vi "BonOMM-SAOMM.vi"() -> ()   [LabVIEW 2019] (continued)
            n4636 = call "PRAMMS-LISTENER.vi"("PRAMMS-COMM IN"=w2155, "Bool Refnum"=w2145, "MessageTypeArray"=w2152, "Signature"=w2144, "Error IN"=w2154, "ReadTimeOut"=4) -> ("Type"=w2147:string, "ByteArray"=w2151:u8[], "Received?"=w2153:bool)  [unwired: 4 in, 3 out]
            n4637 = flat-sequence {
              tunnel: w2153 -> [w2159]
              tunnel: w2151 -> [w2158]
              tunnel: w2147 -> [w2157]
              tunnel: w2139 -> [w2156]
              frame #0 {
                # "Lit toujours le socket prams et rafraichi l'image s'il s'agît d'une image ..."
                n4638 = case shown="Vrai" w2159 {
                  tunnel: w2157 -> [_ w2162]
                  tunnel: w2158 -> [_ w2161]
                  tunnel: w2156 -> [_ w2160]
                  frame False {
                  }
                  frame True {
                    n4639 = case shown="\"emtTelescopeServoLevel\"" w2162 {
                      selector: w2162 -> [w2164 _ _ _ _ _ _ _ _ _ _ _ _ _ _ _ _ _ _ _ _ _ _ w2454 _]
                      tunnel: w2161 -> [w2163 w2176 _ _ _ w2201 w2209 w2236 w2255 w2259 w2263 w2284 w2304 w2309 w2316 w2321 w2328 w2335 _ _ w2350 w2356 w2415 w2451 w2475]
                      tunnel: w2160 -> [_ _ _ _ _ _ _ _ _ _ _ _ _ _ _ _ _ _ _ _ _ _ _ _ w2463]
                      frame "Unknown", Default {
                        w2167 = "\r"
                        n4640 = Type Cast(type=w2167, x=w2163) -> (*(type *) &x=w2166:string)
                        n4641 = local read "Dump"() -> (w2169:string)
                        n4642 = Concatenate Strings(w2169, w2164, " : " ("string"), w2166, w2167) -> (→"Dump":string)
                      }
                      frame "emtError" {
                        # "Tableau d'exception qui ne causeront\npas l'affichage d'un message d'erreur."
                        n4643 = To Unsigned Long Integer(number=u32 0) -> (unsigned 32bit integer=w2178:u32)
                        n4644 = call-poly "SAOMM-EXTRACT-DATA.vi"("UINT32"=w2178, "Data"=w2176) -> ("Value"=w2173:u32)  [unwired: 10 in, 3 out]
                        n4645 = Search 1D Array(1D array=u32[] [64], element=w2173) -> (index of element=w2170:i32)  [unwired: 1 in]
                        n4646 = Less Than 0?(x=w2170) -> (x < 0?=w2171:bool)
                        n4647 = case shown="Vrai" w2171 {
                          tunnel: w2173 -> [_ w2182]
                          frame False {
                          }
                          frame True {
                            n4648 = Not Equal To 0?(x=w2182) -> (x != 0?=w2186:bool)
                            n4649 = case shown="Faux" w2186 {
                              tunnel: w2182 -> [_ w2193]
                              tunnel: ["Erreur reçu de PrAMS (code : indéfini)" w2189] -> w2187
                              frame False {
                              }
                              frame True {
                                n4650 = Number To Decimal String(number=w2193) -> (decimal integer string=w2192:string)  [unwired: 1 in]
                                n4651 = Concatenate Strings("Erreur reçu de PrAMS (code : ", w2192, ")") -> (w2189:string)
                              }
                            }
                            n4652 = local read "FIFO d'erreur"() -> (w2183:T7)
                            n4653 = call "Error_Format.vi"("FIFO IN"=w2183, "Error Code IN"=w2182, "Source"="PrAMS", "Comment"=w2187) -> ("FIFO OUT"=w2184:T7)  [unwired: 13 in, 2 out]
                            n4654 = local write "FIFO d'erreur"(w2184) -> ()
                          }
                        }
                        n4655 = To Long Integer(number=w2173) -> (32bit integer=w2174:i32)
                        n4656 = Negate(x=w2174) -> (-x=w2175:i32)
                        n4657 = local write "PrAMS-ACK"(w2175) -> ()
                        n4658 = local read "Nb_Error (PrAMS)"() -> (w2180:i32)
                        n4659 = Increment(x=w2180) -> (x+1=w2179:i32)
                        n4660 = local write "Nb_Error (PrAMS)"(w2179) -> ()
                        "PrAMS-Error" <- TRUE ("PrAMS-Error")
                      }
                      frame "emtAreYouThere" {
                      }
                      frame "emtAcknowledgment" {
                        n4661 = local read "Nb_ACK (PrAMS)"() -> (w2195:i32)
                        n4662 = Increment(x=w2195) -> (x+1=→"Nb_ACK (PrAMS)":i32)
                        "PrAMS-ACK" <- 1 ("PrAMS-ACK")
                      }
                      frame "emtClientType" {
                        # "Jamais reçu par BonOMM actuellement puisque BonOMM n'envoit pas de \"emtGetClientType\"\n\nEn fait, peut-être qu'il manque un \"Set\" dans l'enum ... genre \"emtSetClientType\""
                      }
                      frame "emtImageExposureTime" {
                        n4663 = To Unsigned Long Integer(number=u32 0) -> (unsigned 32bit integer=w2200:u32)
                        n4664 = call-poly "SAOMM-EXTRACT-DATA.vi"("UINT32"=w2200, "Data"=w2201) -> ("Value"=w2199:u32)  [unwired: 10 in, 3 out]
                        n4665 = To Double Precision Float(number=w2199) -> (double precision float=w2198:dbl)
                        n4666 = expression code="x/1000."(w2198) -> (w2197:dbl)
                        n4667 = local write "exptime"(w2197) -> ()
                      }
                      frame "emtOptimalExposureTime" {
                        n4668 = flat-sequence {
                          tunnel: w2209 -> [w2215]
                          tunnel: [w2212] -> w2207
                          tunnel: [w2211] -> w2205
                          tunnel: [w2210] -> w2203
                          tunnel: [w2222] -> w2208
                          tunnel: w2207 -> [w2222]
                          tunnel: [w2221] -> w2206
                          tunnel: w2205 -> [w2221]
                          tunnel: [w2220] -> w2204
                          tunnel: w2203 -> [w2220]
                          tunnel: w2208 -> [w2228]
                          tunnel: w2206 -> [w2227]
                          tunnel: w2204 -> [w2226]
                          frame #0 {
                            n4669 = To Unsigned Long Integer(number=u32 0) -> (unsigned 32bit integer=w2218:u32)
                            n4670 = call-poly "SAOMM-EXTRACT-DATA.vi"("UINT32"=w2218, "Data"=w2215) -> ("Value"=w2217:u32)  [unwired: 10 in, 3 out]
                            n4671 = To Double Precision Float(number=w2217) -> (double precision float=w2216:dbl)
                            n4672 = expression code="x/1000."(w2216) -> (w2211:dbl)
                            n4673 = In Range and Coerce(upper limit=30.0, x=w2211, lower limit=0.0) -> (coerced(x)=w2210:dbl, In Range?=w2212:bool)
                          }
                          frame #1 {
                            n4674 = local read "GetOptimalTime"() -> (w2224:u32)
                            n4675 = Tick Count (ms)() -> (millisecond timer value=w2223:u32)
                            n4676 = Subtract(x=w2223, y=w2224) -> (x-y=w2225:u32)
                            n4677 = local write "GetOptimalTime"(w2225) -> ()
                          }
                          frame #2 {
                            n4678 = case shown="Vrai" w2228 {
                              tunnel: w2227 -> [w2229 _]
                              tunnel: w2226 -> [_ w2235]
                              frame False {
                                n4679 = Number To Fractional String(number=w2229, precision (6)=i16 2) -> (F-format string=w2233:string)  [unwired: 2 in]
                                n4680 = Concatenate Strings("La valeur optimale retournée (", w2233, ") est hors de l'intervalle acceptée.") -> (w2230:string)
                                n4681 = One Button Dialog(message=w2230) -> ()  [unwired: 1 in, 1 out]
                              }
                              frame True {
                                # "On envoit la nouvelle valeur comme valeur actuelle"
                                n4682 = property on="exptime" class="NumNb (strict)"("Val(Sgnl)"=w2235) -> ()  [unwired: 2 in, 2 out]
                              }
                            }
                          }
                        }
                      }
                      frame "emtImageEMGain" {
                        n4683 = flat-sequence {
                          tunnel: w2236 -> [w2238]
                          frame #0 {
                            n4684 = To Unsigned Word Integer(number=u16 0) -> (unsigned 16bit integer=w2239:u16)
                            n4685 = call-poly "SAOMM-EXTRACT-DATA.vi"("UINT16"=w2239, "Data"=w2238) -> ("Value"=→"EMGain":u16)  [unwired: 10 in, 3 out]
                          }
                          frame #1 {
                            n4686 = local read "QueryingPraMS"() -> (w2241:bool)
                            n4687 = case shown="Vrai" w2241 {
                              frame False {
                              }
                              frame True {
                                n4688 = local read "FalconQuery"() -> (w2244:u32)
                                n4689 = Tick Count (ms)() -> (millisecond timer value=w2245:u32)
                                n4690 = Subtract(x=w2245, y=w2244) -> (x-y=w2243:u32)
                                n4691 = local write "QueryingPraMS"(FALSE ("Querying")) -> ()
                                n4692 = local write "FalconQuery"(w2243) -> ()
                              }
                            }
                          }
                        }
                      }
                      frame "emtFPGACtrl" {
                        n4693 = To Unsigned Word Integer(number=u16 0) -> (unsigned 16bit integer=w2253:u16)
                        n4694 = call-poly "SAOMM-EXTRACT-DATA.vi"("UINT16"=w2253, "Data"=w2255) -> ("Value"=w2247:u16)  [unwired: 10 in, 3 out]
                        "FPGA Value" <- w2247
                        n4695 = Number To Decimal String(number=w2247) -> (decimal integer string=w2250:string)  [unwired: 1 in]
                        n4696 = control-ref of="TERMINAL"() -> (w2251:refnum<vi>)
                        n4697 = control-ref of="Indicateur d'état"() -> (w2252:refnum<vi>)
                        n4698 = Concatenate Strings("FAPG.get -> (", w2250, ")" ("string")) -> (w2246:string)
                        n4699 = call "TERMINAL.vi"("Indicateur Refnum"=w2252, "Terminal Refnum"=w2251, "Indicateur d'état"=w2246) -> ()
                      }
                      frame "emtImageWidth" {
                        n4700 = To Unsigned Word Integer(number=u16 0) -> (unsigned 16bit integer=w2256:u16)
                        n4701 = call-poly "SAOMM-EXTRACT-DATA.vi"("UINT16"=w2256, "Data"=w2259) -> ("Value"=w2258:u16)  [unwired: 10 in, 3 out]
                        n4702 = local write "ImageWidth"(w2258) -> ()
                      }
                      frame "emtImageHeight" {
                        n4703 = To Unsigned Word Integer(number=u16 0) -> (unsigned 16bit integer=w2260:u16)
                        n4704 = call-poly "SAOMM-EXTRACT-DATA.vi"("UINT16"=w2260, "Data"=w2263) -> ("Value"=w2262:u16)  [unwired: 10 in, 3 out]
                        n4705 = local write "ImageHeight"(w2262) -> ()
                      }
                      frame "emtImageBinning" {
                        w2274 = "cam_Binning "
                        n4706 = To Unsigned Word Integer(number=0) -> (unsigned 16bit integer=w2282:u16)
                        n4707 = call-poly "SAOMM-EXTRACT-DATA.vi"("UINT16"=w2282, "Data"=w2284) -> ("Value"=w2269:u16)  [unwired: 10 in, 3 out]
                        n4708 = local write "Binning"(w2269) -> ()
                        n4709 = case shown="1, Par défaut" w2269 {
                          tunnel: [TRUE FALSE FALSE FALSE] -> w2268
                          tunnel: [FALSE TRUE FALSE FALSE] -> w2267
                          tunnel: [FALSE FALSE TRUE FALSE] -> w2266
                          tunnel: [FALSE FALSE FALSE TRUE] -> w2265
                          frame 1, Default {
                          }
                          frame 2 {
                          }
                          frame 4 {
                          }
                          frame 5 {
                          }
                        }
                        n4710 = Current VI's Menubar() -> (w2264:refnum<k9>)
                        n4711 = Concatenate Strings(w2274, "1x1" ("string")) -> (w2273:string)
                        n4712 = Set Menu Item Info(6:w2268, 7:w2273, 11:w2264) -> (3:w2270:refnum<k9>)  [unwired: 4 in, 1 out]
                        n4713 = Concatenate Strings(w2274, "2x2" ("string")) -> (w2279:string)
                        n4714 = Set Menu Item Info(6:w2267, 7:w2279, 11:w2270) -> (3:w2271:refnum<k9>)  [unwired: 4 in, 1 out]
                        n4715 = Concatenate Strings(w2274, "4x4" ("string")) -> (w2280:string)
                        n4716 = Set Menu Item Info(6:w2266, 7:w2280, 11:w2271) -> (3:w2272:refnum<k9>)  [unwired: 4 in, 1 out]
                        n4717 = Concatenate Strings(w2274, "5x5" ("string")) -> (w2281:string)
                        n4718 = Set Menu Item Info(6:w2265, 7:w2281, 11:w2272) -> ()  [unwired: 4 in, 2 out]
                      }
                      frame "emtImageDisplayFrameRate" {
                        n4719 = To Double Precision Float(number=0.0) -> (double precision float=w2302:dbl)
                        n4720 = call-poly "SAOMM-EXTRACT-DATA.vi"("DBL"=w2302, "Data"=w2304) -> ("Value"=w2301:dbl)  [unwired: 10 in, 3 out]
                        n4721 = local write "ImageFPS"(w2301) -> ()
                      }
                      frame "emtROIWidth" {
                        n4722 = To Unsigned Word Integer(number=u16 0) -> (unsigned 16bit integer=w2307:u16)
                        n4723 = call-poly "SAOMM-EXTRACT-DATA.vi"("UINT16"=w2307, "Data"=w2309) -> ("Value"=w2308:u16, "Min"=→"ROIWidthMin":u16, "Max"=→"ROIWidthMax":u16)  [unwired: 10 in, 1 out]
                        n4724 = local write "ROIWidth"(w2308) -> ()
                      }
                      frame "emtROIHeight" {
                        n4725 = To Unsigned Word Integer(number=u16 0) -> (unsigned 16bit integer=w2313:u16)
                        n4726 = call-poly "SAOMM-EXTRACT-DATA.vi"("UINT16"=w2313, "Data"=w2316) -> ("Value"=w2315:u16, "Min"=→"ROIHeightMin":u16, "Max"=→"ROIHeightMax":u16)  [unwired: 10 in, 1 out]
                        n4727 = local write "ROIHeight"(w2315) -> ()
                      }
                      frame "emtROIXOffset" {
                        n4728 = To Unsigned Word Integer(number=u16 0) -> (unsigned 16bit integer=w2319:u16)
                        n4729 = call-poly "SAOMM-EXTRACT-DATA.vi"("UINT16"=w2319, "Data"=w2321) -> ("Value"=w2320:u16, "Min"=w2318:u16, "Max"=w2317:u16)  [unwired: 10 in, 1 out]
                        n4730 = local write "ROIXOffset"(w2320) -> ()
                        n4731 = local write "ROIXMin"(w2318) -> ()
                        n4732 = local write "ROIXMax"(w2317) -> ()
                      }
                      frame "emtROIYOffset" {
                        n4733 = To Unsigned Word Integer(number=u16 0) -> (unsigned 16bit integer=w2325:u16)
                        n4734 = call-poly "SAOMM-EXTRACT-DATA.vi"("UINT16"=w2325, "Data"=w2328) -> ("Value"=w2326:u16, "Min"=w2324:u16, "Max"=w2323:u16)  [unwired: 10 in, 1 out]
                        n4735 = local write "ROIYOffset"(w2326) -> ()
                        n4736 = local write "ROIYMax"(w2323) -> ()
                        n4737 = local write "ROIYMin"(w2324) -> ()
                      }
                      frame "emtTelescopeServoLevel" {
                        # "En supposant que ça retourne le TelescopeServoLevel"
                        # "Si Level > \"Opération Fixe\"\nAlors c'est que l'asservissement\nest enclenché."
                        # "Reçoit la nouvelle valeur de emtTelescopeServoLevel"
                        n4738 = To Unsigned Long Integer(number=0) -> (unsigned 32bit integer=w2333:u32)
                        n4739 = call-poly "SAOMM-EXTRACT-DATA.vi"("UINT32"=w2333, "Data"=w2335) -> ("Value"=w2332:u32)  [unwired: 10 in, 3 out]
                        n4740 = To Unsigned Word Integer(number=w2332) -> (unsigned 16bit integer=w2331:u16)
                        n4741 = Greater?(x=w2331, y=u16 0) -> (0:w2329:bool)
                        n4742 = local write "Mode"(w2331) -> ()
                        n4743 = local write "Servo"(w2329) -> ()
                        n4744 = case shown="Vrai" w2329 {
                          frame False {
                            # "Réinitialise les variables relatives à l'asservissement\nHistorique, etc ..."
                          }
                          frame True {
                          }
                        }
                      }
                      frame "emtAcquisitionStarted" {
                        w2336 = T17."Enabled" ("Disabled")
                        n4745 = local write "Integrating"(TRUE) -> ()
                        n4746 = property on="Mode" class="MDér (strict)"("DisabledEnum"=w2336) -> ()  [unwired: 2 in, 2 out]
                        n4747 = property on="StartServo" class="Bool (strict)"("DisabledEnum"=w2336) -> ()  [unwired: 2 in, 2 out]
                        n4748 = property on="StopServo" class="Bool (strict)"("DisabledEnum"=w2336) -> ()  [unwired: 2 in, 2 out]
                      }
                      frame "emtAcquisitionStopped" {
                        w2339 = FALSE ("Visible")
                        w2340 = "N/D"
                        w2341 = T17."Disabled and Grayed Out" ("Disabled")
                        w2342 = u16 2 items=["Region d'intérêt", "Prévisualisation", "Idle"] ("ImageUsage")
                        n4749 = property on="Mode" class="MDér (strict)"("DisabledEnum"=T17."Enabled" ("Disabled")) -> ()  [unwired: 2 in, 2 out]
                        n4750 = property on="StartServo" class="Bool (strict)"("DisabledEnum"=w2341) -> ()  [unwired: 2 in, 2 out]
                        n4751 = property on="StopServo" class="Bool (strict)"("DisabledEnum"=w2341) -> ()  [unwired: 2 in, 2 out]
                        n4752 = local write "ImageUsage"(w2342) -> ()
                        n4753 = local write "subimg"(sgl[][] [] ("ImgArray")) -> ()
                        n4754 = local write "Integrating"(FALSE) -> ()
                        n4755 = local write "InstantFPS"(0.0 ("InstantFPS")) -> ()
                        n4756 = property on="LowSNR" class="Bool (strict)"("Visible"=w2339, "Blinking"=w2339) -> ()  [unwired: 2 in, 2 out]
                        n4757 = property on="Saturé" class="Bool (strict)"("Visible"=w2339, "Blinking"=w2339) -> ()  [unwired: 2 in, 2 out]
                        "ImgArray" <- u32[][] [] ("ImgArray")
                        "ErrY" <- w2340
                        "ErrX" <- w2340
                      }
                      frame "emtTelescopeServoLevelChanged" {
                        # "Update la nouvelle valeur pour assurer que c'est le bon."
                        n4758 = local read "Mode"() -> (w2349:u16)
                        n4759 = call-poly "SAOMM-EXTRACT-DATA.vi"("UINT16"=w2349, "Data"=w2350) -> ("Value"=w2347:u16)  [unwired: 10 in, 3 out]
                        n4760 = local write "Mode"(w2347) -> ()
                        n4761 = Greater Than 0?(x=w2347) -> (x > 0?=→"Servo":bool)
                      }
                      frame "emtFalconImage" {
                        n4762 = flat-sequence {
                          tunnel: w2356 -> [w2361]
                          tunnel: [w2361] -> w2355
                          tunnel: [w2360] -> w2353
                          tunnel: [w2358] -> w2352
                          tunnel: [w2357] -> w2351
                          tunnel: w2355 -> [w2383]
                          tunnel: [w2377] -> w2354
                          tunnel: w2353 -> [w2377]
                          tunnel: w2352 -> [w2374]
                          tunnel: w2351 -> [w2373]
                          tunnel: w2354 -> [w2414]
                          frame #0 {
                            n4763 = local read "LastImageID"() -> (w2358:u32)
                            n4764 = local write "Integrating"(TRUE) -> ()
                            n4765 = Get Date/Time In Seconds() -> (seconds since 1Jan1904=w2357:timestamp)
                            n4766 = Tick Count (ms)() -> (millisecond timer value=w2360:u32)
                          }
                          frame #1 {
                            # "Comme il n'y a pas de critères sur le ID, il se peut qu'on recoive la dernière image et non la prochaine ..."
                            n4767 = To Double Precision Float(number=w2373) -> (double precision float=w2366:dbl)
                            n4768 = call "PRAMMS-DataString2Image.vi"("ImageData"=w2383) -> ("Width"=→"ImageWidth":u16, "Height"=→"ImageHeight":u16, "Image"=w2363:u16[][], "ImageID"=w2362:u32)  [unwired: 8 in, 3 out]
                            n4769 = local read "LastImageTime"() -> (w2367:dbl)
                            n4770 = local read "SaveNextImage"() -> (w2365:bool)
                            n4771 = To Unsigned Long Integer(number=w2363) -> (unsigned 32bit integer=w2364:u32[][])
                            n4772 = local write "LastImageID"(w2362) -> ()
                            n4773 = local write "ImgArray"(w2364) -> ()
                            n4774 = local read "TmpFalcon"() -> (w2382:u32)
                            n4775 = case shown="Vrai" w2365 {
                              tunnel: w2363 -> [_ w2406]
                              frame False {
                              }
                              frame True {
                                n4776 = Get Date/Time In Seconds() -> (seconds since 1Jan1904=w2396:timestamp)
                                n4777 = local read "path_data"() -> (w2401:path)
                                n4778 = To Double Precision Float(number=w2396) -> (double precision float=w2395:dbl)
                                n4779 = local write "SaveNextImage"(FALSE ("SaveNextImage")) -> ()
                                n4780 = call "GetPathFromTimeStamp.vi"("UTC Time"=FALSE, "LocalTimeStamp"=w2395, "Changement de date à midi ?"=FALSE) -> ("Date String"=w2400:string, "Time String"=w2399:string)  [unwired: 11 in]
                                n4781 = Concatenate Strings(w2400, w2399, ".fits" ("string")) -> (w2397:string)
                                n4782 = Build Path(base path=w2401, name or relative path=path "CameraImages") -> (appended path=w2403:path)
                                n4783 = local read "Dec Sonde"() -> (w2390:dbl)
                                n4784 = local read "ROIYOffset"() -> (w2387:u16)
                                n4785 = local read "Epoch Tel"() -> (w2389:dbl)
                                n4786 = local read "RA Sonde"() -> (w2391:dbl)
                                n4787 = local read "PixScale2"() -> (w2385:dbl)
                                n4788 = local read "ROIXOffset"() -> (w2386:u16)
                                n4789 = local read "exptime"() -> (w2392:dbl)
                                n4790 = local read "PixScale1"() -> (w2384:dbl)
                                n4791 = local read "Binning"() -> (w2388:u16)
                                n4792 = Build Path(base path=w2403, name or relative path=w2397) -> (appended path=w2404:path)
                                n4793 = call "SaveFalconImage.vi"("SavePath"=w2404, "Binning"=w2388, "ROIYOffset"=w2387, "ROIXOffset"=w2386, "PixScale1"=w2384, "Image"=w2406, "EXPTIME"=w2392, "RA Sonde"=w2391, "Dec Sonde"=w2390, "Epoch Tel"=w2389, "PixScale2"=w2385) -> ()  [unwired: 5 in]
                              }
                            }
                            n4794 = Subtract(x=w2366, y=w2367) -> (x-y=w2370:dbl)
                            n4795 = Greater?(x=w2362, y=w2374) -> (0:w2372:bool)
                            n4796 = Tick Count (ms)() -> (millisecond timer value=w2381:u32)
                            n4797 = flat-sequence {
                              tunnel: w2382 -> [w2411]
                              tunnel: w2381 -> [w2410]
                              tunnel: [w2409] -> w2380
                              frame #0 {
                                n4798 = Subtract(x=w2410, y=w2411) -> (x-y=w2409:u32)
                                "TmpFalcon" <- w2410
                              }
                            }
                            n4799 = Greater?(x=w2370, y=0.5) -> (0:w2368:bool)
                            n4800 = And(x=w2372, y=w2368) -> (x .and. y?=w2371:bool)
                            n4801 = To Double Precision Float(number=w2380) -> (double precision float=w2379:dbl)
                            n4802 = case shown="Vrai" w2371 {
                              selector: w2371 -> [_ w2408]
                              tunnel: w2366 -> [_ w2407]
                              frame False {
                              }
                              frame True {
                                n4803 = property on="FalconProcessed" class="Bool (strict)"("Val(Sgnl)"=w2408) -> ()  [unwired: 2 in, 2 out]
                                "LastImageTime" <- w2407
                              }
                            }
                            n4804 = expression code="1/(x/1000)"(w2379) -> (→"InstantFPS":dbl)
                          }
                          frame #2 {
                            n4805 = Tick Count (ms)() -> (millisecond timer value=w2413:u32)
                            n4806 = Subtract(x=w2413, y=w2414) -> (x-y=→"ImageProcessing":u32)
                          }
                        }
                      }
                      frame "emtProcessedFalconImage" {
                        n4807 = flat-sequence {
                          tunnel: w2415 -> [w2419]
                          frame #0 {
                            w2443 = u16 0 items=["Region d'intérêt", "Prévisualisation"] ("ImageUsage")
                            # "Devrais peut-être servir uniquement à recevoir la sous-image ..."
                            # "Viens pluôt de FalconImage"
                            # "Vérifier le format ..."
                            # "Possiblement ajouter/soustraire 0.5 pixels ..."
                            n4808 = call "SAOMM-ProcImageParser.vi"("ProcessedData"=w2419) -> ("ImageBuffer"=→"ImageBuffer":u16[][], "GrayLevels"=w2417:u8[][], "MaskObjet"=→"MaskObjet":u8[][], "GeneralProperties"=w2428:T54, "ROIProperties"=w2429:T55, "ProcessedProperties"=w2444:T56)  [unwired: 8 in, 1 out]
                            n4809 = Unbundle By Name(w2429) -> ("Position X de la ROI"=w2427:u16)
                            n4810 = Unbundle By Name(w2429) -> ("Position Y de la ROI"=w2425:u16)
                            n4811 = Unbundle By Name(w2444) -> ("Centroide X"=w2426:dbl)
                            n4812 = Unbundle By Name(w2429) -> ("Hauteur de la ROI"=w2441:u16)
                            n4813 = Unbundle By Name(w2444) -> ("Centroide Y"=w2424:dbl)
                            n4814 = Unbundle By Name(w2429) -> ("Largeur de la ROI"=w2442:u16)
                            n4815 = local read "Nb_FalconProc_reçu"() -> (w2422:u32)
                            n4816 = To Single Precision Float(number=w2417) -> (single precision float=w2447:sgl[][])
                            n4817 = Array Max & Min(array=w2447) -> (max value=w2445:sgl)  [unwired: 3 out]
                            n4818 = call "Draw_crosshair.vi"("Image IN"=w2447, "White Value"=w2445) -> ("Image OUT"=w2446:sgl[][])  [unwired: 13 in]
                            n4819 = local write "ROIWidth"(w2442) -> ()
                            n4820 = local write "ROIHeight"(w2441) -> ()
                            n4821 = To Double Precision Float(number=w2427) -> (double precision float=w2435:dbl)
                            n4822 = To Double Precision Float(number=w2425) -> (double precision float=w2434:dbl)
                            n4823 = Increment(x=w2422) -> (x+1=→"Nb_FalconProc_reçu":u32)
                            n4824 = local write "subimg"(w2446) -> ()
                            n4825 = Add(x=w2426, y=w2435) -> (x+y=w2432:dbl)
                            "XCentroid" <- w2432
                            n4826 = Add(x=w2434, y=w2424) -> (x+y=w2433:dbl)
                            "YCentroid" <- w2433
                            n4827 = local read "XReference"() -> (w2431:dbl)
                            n4828 = local write "ROIXOffset"(w2427) -> ()
                            n4829 = local read "YReference"() -> (w2430:dbl)
                            n4830 = local write "ROIYOffset"(w2425) -> ()
                            n4831 = Unbundle By Name(w2428) -> ("ID de l'image"=w2436:u32)
                            n4832 = Subtract(x=w2431, y=w2432) -> (x-y=w2420:dbl)
                            "DiffX" <- w2420
                            n4833 = Subtract(x=w2430, y=w2433) -> (x-y=w2421:dbl)
                            "DiffY" <- w2421
                            n4834 = local write "LastProcID"(w2436) -> ()
                            n4835 = Number To Fractional String(number=w2421, precision (6)=i16 1) -> (F-format string=w2437:string)  [unwired: 2 in]
                            n4836 = Number To Fractional String(number=w2420, precision (6)=i16 1) -> (F-format string=w2438:string)  [unwired: 2 in]
                            n4837 = local write "ErrY"(w2437) -> ()
                            n4838 = local write "ErrX"(w2438) -> ()
                            "ImageUsage" <- w2443
                            "FalconProcData" <- w2419
                          }
                          frame #1 {
                            # "Certaines images entrent après la réception d'un\nacquisition stopped ..."
                            n4839 = local read "Integrating"() -> (w2448:bool)
                            n4840 = case shown="Vrai" w2448 {
                              frame False {
                              }
                              frame True {
                                n4841 = property on="ProcessImage" class="Bool (strict)"("Val(Sgnl)"=TRUE ("Value (Signaling)")) -> ()  [unwired: 2 in, 2 out]
                              }
                            }
                          }
                        }
                      }
                      frame "emtROIXReferencePoint", "emtROIYReferencePoint" {
                        n4842 = To Double Precision Float(number=u16 0) -> (double precision float=w2452:dbl)
                        n4843 = call-poly "SAOMM-EXTRACT-DATA.vi"("DBL"=w2452, "Data"=w2451) -> ("Value"=w2450:dbl)  [unwired: 10 in, 3 out]
                        n4844 = case shown="\"emtROIXReferencePoint\"" w2454 {
                          tunnel: w2450 -> [_ w2456 w2462]
                          frame Default {
                          }
                          frame "emtROIXReferencePoint" {
                            n4845 = local read "ROIXOffset"() -> (w2458:u16)
                            n4846 = To Double Precision Float(number=w2458) -> (double precision float=w2457:dbl)
                            n4847 = Add(x=w2457, y=w2456) -> (x+y=w2455:dbl)
                            n4848 = local write "XReference"(w2455) -> ()
                            "XROIRef" <- w2456
                          }
                          frame "emtROIYReferencePoint" {
                            n4849 = local read "ROIYOffset"() -> (w2461:u16)
                            n4850 = To Double Precision Float(number=w2461) -> (double precision float=w2460:dbl)
                            n4851 = Add(x=w2460, y=w2462) -> (x+y=w2459:dbl)
                            n4852 = local write "YReference"(w2459) -> ()
                            "YROIRef" <- w2462
                          }
                        }
                      }
                      frame "emtHexapodServoCommandLogging" {
                        # "Nombre de secondes entre les\npremiers janvier 1904 et 1970"
                        # "Utilisation des éléments de HexapodServoCommandLogging"
                        n4853 = call "SAOMM-HistoParser.vi"("DataStream"=w2475) -> ("Source cluster"=w2469:T57, "Hexapod cluster"=w2474:T58)  [unwired: 13 in]
                        n4854 = local read "ConsideredLenght"() -> (w2473:i32)
                        n4855 = Unbundle By Name(w2469) -> ("Logging TimeStapmp"=w2467:u64)
                        n4856 = To Double Precision Float(number=w2467) -> (double precision float=w2468:dbl)
                        n4857 = Unbundle By Name(w2469) -> ("SNR"=w2471:dbl)
                        n4858 = expression code="x/1000"(w2468) -> (w2466:dbl)
                        n4859 = To Double Precision Float(number=w2473) -> (double precision float=w2472:dbl)
                        n4860 = Add(x=w2466, y=2082844799.0) -> (x+y=w2464:dbl)
                        n4861 = local write "LoggingTimeStamp"(w2464) -> ()
                        n4862 = Not Equal To 0?(x=w2471) -> (x != 0?=w2470:bool)
                        n4863 = case shown="Vrai" w2470 {
                          tunnel: w2474 -> [_ w2480]
                          tunnel: w2472 -> [_ w2479]
                          tunnel: w2469 -> [_ w2478]
                          tunnel: w2464 -> [_ w2477]
                          tunnel: w2463 -> [_ w2476]
                          frame False {
                          }
                          frame True {
                            n4864 = stacked-sequence {
                              tunnel: w2480 -> [w2540 _ _ w2635]
                              tunnel: w2478 -> [w2545 _ w2574 _]
                              tunnel: w2479 -> [_ _ w2573 w2634]
                              tunnel: [w2509 _ _ _] -> _
                              tunnel: w2477 -> [_ _ w2558 w2628]
                              tunnel: w2476 -> [_ _ _ _]
                              frame #0 {
                                # "Update des valeurs associées à la trame ..."
                                n4865 = Unbundle By Name(w2540) -> ("Hexapod_Nominal"=w2539:dbl[], "Hexapod_Offset"=w2528:dbl[], "Hexapod_LUT"=w2527:dbl[], "Hexapod_ServoX"=w2525:dbl[], "Hexapode_ServoY"=w2524:dbl[], "Hexapod_Console"=→"H_Console":dbl[], "Hexapod_Position"=w2514:dbl[], "Hexapod_Command"=w2520:dbl[])  [unwired: 1 out]
                                "H_Offset" <- w2528
                                "H_LUT" <- w2527
                                "H_Position" <- w2514
                                "H_Command" <- w2520
                                n4866 = Unbundle By Name(w2545) -> ("ServoLevel"=w2509:u16, "ROIXOffset"=w2544:u16, "ROIYOffset"=w2542:u16, "Pixel X"=w2511:dbl, "Pixel Y"=w2513:dbl, "Flux"=w2485:dbl, "SNR"=w2484:dbl, "CentroidX"=w2543:dbl, "CentroidY"=w2541:dbl, "SNRTreshold"=w2483:dbl)
                                "Flux inst." <- w2485
                                n4867 = Greater Or Equal?(x=w2484, y=w2483) -> (x >= y?=w2482:bool)
                                n4868 = Not(x=w2482) -> (.not. x?=w2481:bool)
                                n4869 = Index Array(array=w2524) -> (element=w2522:dbl)  [unwired: 1 in]
                                n4870 = Index Array(array=w2525) -> (element=w2523:dbl)  [unwired: 1 in]
                                n4871 = local write "SNR"(w2484) -> ()
                                n4872 = Build Array(w2523, w2522) -> (→"H_Servo":dbl[])
                                n4873 = property on="LowSNR" class="Bool (strict)"("Visible"=w2481, "Blinking"=w2481) -> ()  [unwired: 2 in, 2 out]
                                n4874 = Index Array(array=w2539) -> (element #1=→"Nominal X":dbl, element #2=→"Nominal Y":dbl, element #3=→"Nominal Z":dbl, element #4=→"Nominal U":dbl, element #5=→"Nominal V":dbl, element #6=→"Nominal W":dbl)  [unwired: 6 in]
                                n4875 = local write "ROIYOffset"(w2542) -> ()
                                n4876 = Index Array(array=w2527) -> (element #1=→"LUT X":dbl, element #2=→"LUT Y":dbl, element #3=→"LUT Z":dbl, element #4=→"LUT U":dbl, element #5=→"LUT V":dbl, element #6=→"LUT W":dbl)  [unwired: 6 in]
                                n4877 = local write "YROIRef"(w2513) -> ()
                                n4878 = local write "ROIXOffset"(w2544) -> ()
                                n4879 = local write "XROIRef"(w2511) -> ()
                                n4880 = local read "Flux Max"() -> (w2488:dbl)
                                n4881 = local read "Flux Min"() -> (w2487:dbl)
                                n4882 = Index Array(array=w2528) -> (element #1=w2538:dbl, element #2=w2537:dbl, element #3=w2536:dbl, element #4=w2535:dbl, element #5=w2534:dbl)  [unwired: 5 in]
                                n4883 = Greater?(x=w2485, y=w2488) -> (0:w2489:bool)
                                n4884 = Less?(x=w2485, y=w2487) -> (x < y?=w2486:bool)
                                n4885 = Index Array(array=w2514) -> (element #1=→"HexX":dbl, element #2=→"HexY":dbl, element #3=→"HexZ":dbl, element #4=→"HexU":dbl, element #5=→"HexV":dbl, element #6=→"HexW":dbl)  [unwired: 6 in]
                                n4886 = local write "Offset X"(w2538) -> ()
                                n4887 = local write "Offset Y"(w2537) -> ()
                                n4888 = local write "Offset Z"(w2536) -> ()
                                n4889 = local write "Offset U"(w2535) -> ()
                                n4890 = local write "Offset V"(w2534) -> ()
                                n4891 = case shown="Vrai" w2489 {
                                tunnel: w2485 -> [_ w2547]
                                frame False {
                                }
                                frame True {
                                "Flux Max" <- w2547
                                }
                                }
                                n4892 = case shown="Vrai" w2486 {
                                tunnel: w2485 -> [_ w2546]
                                frame False {
                                }
                                frame True {
                                "Flux Min" <- w2546
                                }
                                }
                                n4893 = To Double Precision Float(number=w2544) -> (double precision float=w2510:dbl)
                                n4894 = To Double Precision Float(number=w2542) -> (double precision float=w2512:dbl)
                                n4895 = Add(x=w2510, y=w2543) -> (x+y=w2494:dbl)
                                n4896 = Add(x=w2512, y=w2541) -> (x+y=w2493:dbl)
                                n4897 = local write "XCentroid"(w2494) -> ()
                                n4898 = Add(x=w2510, y=w2511) -> (x+y=w2495:dbl)
                                n4899 = Add(x=w2512, y=w2513) -> (x+y=w2492:dbl)
                                n4900 = Index Array(array=w2520) -> (element #1=→"Cmd X":dbl, element #2=→"Cmd Y":dbl, element #3=→"Cmd Z":dbl, element #4=→"Cmd U":dbl, element #5=→"Cmd V":dbl)  [unwired: 5 in]
                                n4901 = local write "YCentroid"(w2493) -> ()
                                n4902 = local write "XReference"(w2495) -> ()
                                n4903 = local write "YReference"(w2492) -> ()
                                n4904 = Subtract(x=w2495, y=w2494) -> (x-y=w2490:dbl)
                                n4905 = Subtract(x=w2492, y=w2493) -> (x-y=w2491:dbl)
                                n4906 = local write "DiffX"(w2490) -> ()
                                n4907 = local write "DiffY"(w2491) -> ()
                              }
                              frame #1 {
                                # "À terme, il faudra ici que l'écart soit :\n\n- Opération fixe : Hpos - Hoff\n- En boucle ouverte : Hpos - (Hlut + Hoff)\n- En asservissement : Hpos - (HOff)"
                                n4908 = local read "H_Offset"() -> (w2551:dbl[])
                                n4909 = local read "H_LUT"() -> (w2552:dbl[])
                                n4910 = local read "H_Position"() -> (w2553:dbl[])
                                n4911 = Add(x=w2552, y=w2551) -> (x+y=w2550:dbl[])
                                n4912 = Subtract(x=w2553, y=w2550) -> (x-y=w2554:dbl[])
                                n4913 = Index Array(array=w2554) -> (element #1=→"EcartX":dbl, element #2=→"EcartY":dbl, element #3=→"EcartZ":dbl, element #4=→"EcartU":dbl, element #5=→"EcartV":dbl)  [unwired: 5 in]
                              }
                              frame #2 {
                                # "ServoLevel = -1 si inactif ..."
                                # "Update des graphiques de guidage"
                                n4914 = Unbundle By Name(w2574) -> ("ServoLevel"=w2570:u16, "ROIXOffset"=w2580:u16, "CentroidX"=w2581:dbl, "Pixel X"=w2582:dbl, "ROIYOffset"=w2583:u16, "CentroidY"=w2584:dbl, "Pixel Y"=w2585:dbl)
                                n4915 = Unbundle By Name(w2574) -> ("SNR"=w2578:dbl, "SNRTreshold"=w2577:dbl, "Flux"=w2579:dbl)
                                n4916 = local read "Servo"() -> (w2569:bool)
                                n4917 = Boolean To (0,1)(Boolean=w2569) -> (0, 1=w2572:i16)
                                n4918 = Greater Than 0?(x=w2570) -> (x > 0?=w2571:bool)
                                n4919 = local read "CentroidsData"() -> (w2564:cluster{dbl[], dbl[]}[])
                                n4920 = local read "SNRData"() -> (w2563:cluster{dbl[], dbl[]}[])
                                n4921 = local read "FluxData"() -> (w2562:cluster{dbl[], dbl[]}[])
                                n4922 = Decrement(x=w2572) -> (x-1=w2568:i16)
                                n4923 = Bundle("SNR"=w2578, "SNRTreshold"=w2577, "Flux"=w2579) -> (w2575:T59)  [unwired: 1 in]
                                n4924 = To Unsigned Word Integer(number=w2568) -> (unsigned 16bit integer=w2567:u16)
                                n4925 = Select(t=w2570, s=w2571, f=w2567) -> (s? t:f=w2566:u16)
                                n4926 = Bundle("ServoLevel"=w2566, "ROIXOffset"=w2580, "CentroidX"=w2581, "Pixel X"=w2582, "ROIYOffset"=w2583, "CentroidY"=w2584, "Pixel Y"=w2585) -> (w2576:T60)  [unwired: 1 in]
                                n4927 = call "SAOMM-Graph-Guiding.vi"("SNR Data"=w2575, "TimeStamp"=w2558, "DataLenght (seconds)"=w2573, "Centroids Data"=w2576, "SNR IN"=w2563, "Flux IN"=w2562, "Centroids IN"=w2564) -> ("SNR OUT"=w2560:cluster{dbl[], dbl[]}[], "Flux OUT"=w2559:cluster{dbl[], dbl[]}[], "Centroids OUT"=w2561:cluster{dbl[], dbl[]}[])  [unwired: 6 in]
                                "SNRData" <- w2560
                                "FluxData" <- w2559
                                "CentroidsData" <- w2561
                                n4928 = local read "Servo"() -> (w2565:bool)
                                n4929 = case shown="Vrai" w2565 {
                                tunnel: w2560 -> [_ w2622]
                                tunnel: w2559 -> [_ w2620]
                                tunnel: w2561 -> [_ w2625]
                                frame False {
                                }
                                frame True {
                                w2596 = 100.0 ("y")
                                n4930 = local read "GraphTimeStamp"() -> (w2618:dbl)
                                n4931 = Array Subset(array=w2625, index=0, length=2) -> (w2619:cluster{dbl[], dbl[]}[])
                                n4932 = local read "Binning"() -> (w2611:u16)
                                n4933 = local read "PixScale1"() -> (w2610:dbl)
                                n4934 = call "TroncateGraphData.vi"("TimeStampTreshold"=w2618, "Data IN"=w2622) -> ("Truncated Data"=→"Graph-SNR":cluster{dbl[], dbl[]}[])  [unwired: 13 in]
                                n4935 = call "TroncateGraphData.vi"("TimeStampTreshold"=w2618, "Data IN"=w2620) -> ("Truncated Data"=w2601:cluster{dbl[], dbl[]}[])  [unwired: 13 in]
                                n4936 = call "TroncateGraphData.vi"("TimeStampTreshold"=w2618, "Data IN"=w2619) -> ("Truncated Data"=w2617:cluster{dbl[], dbl[]}[])  [unwired: 13 in]
                                n4937 = To Double Precision Float(number=w2611) -> (double precision float=w2612:dbl)
                                n4938 = Index Array(array=w2617) -> (element #1=w2615:cluster{dbl[], dbl[]}, element #2=w2616:cluster{dbl[], dbl[]})  [unwired: 2 in]
                                n4939 = Index Array(array=w2601) -> (element #1=w2594:cluster{dbl[], dbl[]}, element #2=w2595:cluster{dbl[], dbl[]})  [unwired: 2 in]
                                n4940 = Multiply(x=w2612, y=w2610) -> (x*y=w2609:dbl)
                                n4941 = local read "Flux Max"() -> (w2591:dbl)
                                n4942 = Unbundle(w2615) -> (w2607:dbl[], w2614:dbl[])
                                n4943 = Unbundle(w2616) -> (w2608:dbl[], w2613:dbl[])
                                n4944 = Unbundle(w2594) -> (w2598:dbl[], w2593:dbl[])
                                n4945 = Unbundle(w2595) -> (w2597:dbl[], w2592:dbl[])
                                n4946 = Multiply(x=w2614, y=w2609) -> (x*y=w2606:dbl[])
                                n4947 = Multiply(x=w2613, y=w2609) -> (x*y=w2605:dbl[])
                                n4948 = Bundle(w2607, w2606) -> (w2603:cluster{dbl[], dbl[]})  [unwired: 1 in]
                                n4949 = Bundle(w2608, w2605) -> (w2604:cluster{dbl[], dbl[]})  [unwired: 1 in]
                                n4950 = Divide(x=w2593, y=w2591) -> (x/y=w2590:dbl[])
                                n4951 = Divide(x=w2592, y=w2591) -> (x/y=w2589:dbl[])
                                n4952 = Build Array(w2603, w2604) -> (→"Graph-Centroids":cluster{dbl[], dbl[]}[])
                                n4953 = Multiply(x=w2590, y=w2596) -> (x*y=w2599:dbl[])
                                n4954 = Multiply(x=w2589, y=w2596) -> (x*y=w2600:dbl[])
                                n4955 = Bundle(w2598, w2599) -> (w2588:cluster{dbl[], dbl[]})  [unwired: 1 in]
                                n4956 = Bundle(w2597, w2600) -> (w2587:cluster{dbl[], dbl[]})  [unwired: 1 in]
                                n4957 = Build Array(w2588, w2587) -> (→"Graph-Flux":cluster{dbl[], dbl[]}[])
                                }
                                }
                              }
                              frame #3 {
                                # "Update des graphiques de l'hexapode"
                                n4958 = local read "CumulativeError"() -> (w2626:cluster{dbl[], dbl[]}[])
                                n4959 = local read "HexXData"() -> (w2633:cluster{dbl[], dbl[]}[])
                                n4960 = local read "HexYData"() -> (w2632:cluster{dbl[], dbl[]}[])
                                n4961 = call "SAOMM-Graph-Hexapode.vi"("Hexapod cluster"=w2635, "LoggingTimeStamp"=w2628, "DataLenght (seconds)"=w2634, "X IN"=w2633, "Y IN"=w2632, "Cumul IN"=w2626) -> ("X OUT"=w2631:cluster{dbl[], dbl[]}[], "Y OUT"=w2630:cluster{dbl[], dbl[]}[], "Cumul OUT"=w2627:cluster{dbl[], dbl[]}[])  [unwired: 7 in]
                                "HexXData" <- w2631
                                "HexYData" <- w2630
                                "CumulativeError" <- w2627
                                n4962 = local read "Servo"() -> (w2629:bool)
                                n4963 = case shown="Vrai" w2629 {
                                tunnel: w2631 -> [_ w2642]
                                tunnel: w2630 -> [_ w2641]
                                tunnel: w2627 -> [_ w2637]
                                frame False {
                                }
                                frame True {
                                n4964 = local read "GraphTimeStamp"() -> (w2636:dbl)
                                n4965 = call "TroncateGraphData.vi"("TimeStampTreshold"=w2636, "Data IN"=w2642) -> ("Truncated Data"=→"Hex-XGraph":cluster{dbl[], dbl[]}[])  [unwired: 13 in]
                                n4966 = call "TroncateGraphData.vi"("TimeStampTreshold"=w2636, "Data IN"=w2641) -> ("Truncated Data"=→"Hex-YGraph":cluster{dbl[], dbl[]}[])  [unwired: 13 in]
                                n4967 = call "TroncateGraphData.vi"("TimeStampTreshold"=w2636, "Data IN"=w2637) -> ("Truncated Data"=→"Cumulatif":cluster{dbl[], dbl[]}[])  [unwired: 13 in]
                                }
                                }
                              }
                            }
                          }
                        }
                      }
                    }
                  }
                }
              }
              frame #1 {
                n4968 = Wait (ms)(milliseconds to wait=u32 5) -> ()  [unwired: 1 out]
              }
            }
            n4969 = Tick Count (ms)() -> (millisecond timer value=w2150:u32)
            n4970 = Subtract(x=w2150, y=w2149) -> (x-y=→"ListenerExec":u32)
            n4971 = local read "Archivage SAOMM"() -> (w2140:bool)
            n4972 = local read "PrAMS + SAOMM"() -> (w2141:bool)
            n4973 = local read "Quit"() -> (w2142:bool)
            n4974 = Compound Arithmetic op=AND(w2140, w2141, w2142) -> (w2143:bool)
          }
          "PrAMS Listener" <- w974
          n4975 = while {
            shift-right: [w3663] -> _
            shift-left: w986 -> [w3662]
            shift-left: w986 -> [w3661]
            tunnel: [w3648] -> w979
            i -> [w3649]
            stop <- w3648 stop-if-true
            # "Optimisé pour f=5Hz"
            # "Structure de gestion des itérations périodiques"
            n4976 = local read "Hexapod COMM"() -> (w3650:bool)
            n4977 = Subtract(x=w3662, y=w3661) -> (x-y=→"TimeBetweenExec":u32)
            n4978 = local read "ExCmd COMM"() -> (w3654:bool)
            n4979 = local read "PrAMS COMM"() -> (w3653:bool)
            n4980 = local read "Calib COMM"() -> (w3655:bool)
            n4981 = local read "MCB COMM"() -> (w3651:bool)
            n4982 = local read "TCS COMM"() -> (w3652:bool)
            n4983 = local read "TableCOM"() -> (w3656:bool)
            n4984 = local read "MovingZ"() -> (w3657:bool)
            n4985 = local read "MovingXY"() -> (w3658:bool)
            n4986 = stacked-sequence {
              seq-local: [w3664 _ _ _ _ _ _ _ _ _ _ _ _] -> [_ _ _ _ _ _ _ _ _ _ _ w4111 _]
              seq-local: [_ w3693 _ _ _ _ _ _ _ _ _ _ _] -> [_ _ w3756 w3773 _ _ _ _ _ _ _ _ _]
              seq-local: [_ _ w3757 _ _ _ _ _ _ _ _ _ _] -> [_ _ _ _ w3843 _ _ _ _ _ _ _ _]
              seq-local: [_ _ _ w3774 _ _ _ _ _ _ _ _ _] -> [_ _ _ _ _ _ _ _ _ _ _ _ _]
              seq-local: [_ _ _ _ w3844 _ _ _ _ _ _ _ _] -> [_ _ _ _ _ _ w3903 _ _ _ _ _ _]
              seq-local: [_ _ _ _ _ _ w3902 _ _ _ _ _ _] -> [_ _ _ _ _ _ _ _ _ _ w4068 _ _]
              seq-local: [_ _ _ _ _ _ _ _ _ _ w4067 _ _] -> [_ _ _ _ _ _ _ _ _ _ _ _ _]
              seq-local: [_ _ _ _ _ _ _ _ w3911 _ _ _ _] -> [_ _ _ _ _ _ _ _ _ _ _ w4108 _]
              seq-local: [_ _ _ _ _ _ _ w3906 _ _ _ _ _] -> [_ _ _ _ _ _ _ _ w3910 _ _ _ _]
              seq-local: [_ _ _ _ _ _ _ w3905 _ _ _ _ _] -> [_ _ _ _ _ _ _ _ w3909 _ _ _ _]
              seq-local: [_ _ _ _ _ _ _ w3904 _ _ _ _ _] -> [_ _ _ _ _ _ _ _ w3908 _ _ _ _]
              tunnel: w3658 -> [_ _ _ _ _ _ _ _ _ w3950 _ _ _]
              tunnel: w3657 -> [_ _ _ _ _ _ _ _ _ w3946 _ _ _]
              tunnel: w3656 -> [_ w3692 _ _ _ _ _ _ _ _ _ _ _]
              tunnel: w3655 -> [_ w3691 _ _ _ _ _ _ _ _ _ _ _]
              tunnel: w3654 -> [_ w3690 _ _ _ _ _ _ _ _ _ _ _]
              tunnel: w3653 -> [_ w3689 _ _ _ _ _ _ _ _ _ _ _]
              tunnel: w3652 -> [_ w3688 _ _ _ _ _ _ _ _ _ _ _]
              tunnel: w3651 -> [_ w3687 _ _ _ _ _ _ _ _ _ _ _]
              tunnel: w3650 -> [_ w3677 _ _ _ _ _ _ _ _ _ _ _]
              tunnel: w3649 -> [_ w3669 _ _ _ _ _ _ _ _ _ _ _]
              frame #0 {
                n4987 = Tick Count (ms)() -> (millisecond timer value=w3664:u32)
              }
              frame #1 {
                w3676 = "-1" ("y")
                w3699 = "-1" ("y")
                w3702 = "-1" ("y")
                w3703 = "-1" ("y")
                w3706 = "-1" ("y")
                w3707 = "-1" ("y")
                w3711 = "-1" ("y")
                # "Update le menu s'il y a lieu ..."
                # "Vérification des erreurs de communications"
                n4988 = local read "MC-BonOMM VRN"() -> (w3694:refnum<visa-resource-name>)
                n4989 = local read "Hexapod VRN"() -> (w3674:refnum<visa-resource-name>)
                n4990 = local read "PrAMS VRN"() -> (w3696:refnum<visa-resource-name>)
                n4991 = local read "Excmd VRN"() -> (w3697:refnum<visa-resource-name>)
                n4992 = local read "Table VRN"() -> (w3709:refnum<visa-resource-name>)
                n4993 = local read "Calib VRN"() -> (w3698:refnum<visa-resource-name>)
                n4994 = local read "TCS VRN"() -> (w3695:refnum<visa-resource-name>)
                n4995 = Build Array(w3692, w3691, w3690, w3689, w3688, w3687, w3677) -> (w3681:bool[])
                n4996 = Boolean Array To Number(Boolean array=w3681) -> (number=w3678:u32)
                n4997 = Type Cast(type=w3676, x=w3674) -> (*(type *) &x=w3675:string)
                n4998 = Type Cast(type=w3711, x=w3709) -> (*(type *) &x=w3710:string)
                n4999 = Type Cast(type=w3707, x=w3698) -> (*(type *) &x=w3708:string)
                n5000 = Type Cast(type=w3706, x=w3697) -> (*(type *) &x=w3705:string)
                n5001 = Type Cast(type=w3703, x=w3696) -> (*(type *) &x=w3704:string)
                n5002 = Type Cast(type=w3702, x=w3695) -> (*(type *) &x=w3701:string)
                n5003 = Type Cast(type=w3699, x=w3694) -> (*(type *) &x=w3700:string)
                n5004 = Tick Count (ms)() -> (millisecond timer value=w3693:u32)
                n5005 = Not Equal?(x=w3675, y=w3676) -> (x != y?=w3673:bool)
                n5006 = Not Equal?(x=w3710, y=w3711) -> (x != y?=w3672:bool)
                n5007 = Not Equal?(x=w3708, y=w3707) -> (x != y?=w3686:bool)
                n5008 = Not Equal?(x=w3705, y=w3706) -> (x != y?=w3685:bool)
                n5009 = Not Equal?(x=w3704, y=w3703) -> (x != y?=w3684:bool)
                n5010 = Not Equal?(x=w3701, y=w3702) -> (x != y?=w3683:bool)
                n5011 = Not Equal?(x=w3700, y=w3699) -> (x != y?=w3682:bool)
                n5012 = case shown="Faux" w3672 {
                  frame False {
                    n5013 = local write "NeedOrigin"(TRUE ("Blinking")) -> ()
                  }
                  frame True {
                  }
                }
                n5014 = Build Array(w3672, w3686, w3685, w3684, w3683, w3682, w3673) -> (w3680:bool[])
                n5015 = Boolean Array To Number(Boolean array=w3680) -> (number=w3679:u32)
                n5016 = Not Equal?(x=w3679, y=w3678) -> (x != y?=w3671:bool)
                n5017 = Equal To 0?(x=w3669) -> (x = 0?=w3670:bool)
                n5018 = local read "ReconnectionMute"() -> (w3667:bool)
                n5019 = Or(x=w3671, y=w3670) -> (x .or. y?=w3668:bool)
                n5020 = Not(x=w3667) -> (.not. x?=w3666:bool)
                n5021 = And(x=w3666, y=w3668) -> (x .and. y?=w3665:bool)
                n5022 = case shown="Vrai" w3665 {
                  tunnel: w3672 -> [_ w3751]
                  tunnel: w3686 -> [_ w3754]
                  tunnel: w3685 -> [_ w3753]
                  tunnel: w3684 -> [_ w3750]
                  tunnel: w3683 -> [_ w3748]
                  tunnel: w3682 -> [_ w3752]
                  tunnel: w3673 -> [_ w3749]
                  frame False {
                  }
                  frame True {
                    n5023 = Current VI's Menubar() -> (w3747:refnum<k9>)
                    n5024 = local write "TableCOM"(w3751) -> ()
                    n5025 = Set Menu Item Info(6:w3751, 7:"com_Tables de guidage" ("menu tag"), 11:w3747) -> (0:w3745:errorcluster, 3:w3746:refnum<k9>)  [unwired: 4 in]
                    n5026 = local write "Calib COMM"(w3754) -> ()
                    n5027 = Set Menu Item Info(6:w3754, 7:"com_Module de calibration" ("menu tag"), 8:w3745, 11:w3746) -> (0:w3743:errorcluster, 3:w3744:refnum<k9>)  [unwired: 3 in]
                    n5028 = local write "ExCmd COMM"(w3753) -> ()
                    n5029 = Set Menu Item Info(6:w3753, 7:"com_Commandes externes" ("menu tag"), 8:w3743, 11:w3744) -> (0:w3741:errorcluster, 3:w3742:refnum<k9>)  [unwired: 3 in]
                    n5030 = local write "PrAMS COMM"(w3750) -> ()
                    n5031 = Set Menu Item Info(6:w3750, 7:"com_Caméra de référence" ("menu tag"), 8:w3741, 11:w3742) -> (0:w3739:errorcluster, 3:w3740:refnum<k9>)  [unwired: 3 in]
                    n5032 = local write "TCS COMM"(w3748) -> ()
                    n5033 = Set Menu Item Info(6:w3748, 7:"com_Telescope Control System" ("menu tag"), 8:w3739, 11:w3740) -> (0:w3737:errorcluster, 3:w3738:refnum<k9>)  [unwired: 3 in]
                    n5034 = local write "MCB COMM"(w3752) -> ()
                    n5035 = Set Menu Item Info(6:w3752, 7:"com_MC-BonOMM" ("menu tag"), 8:w3737, 11:w3738) -> (0:w3716:errorcluster, 3:w3717:refnum<k9>)  [unwired: 3 in]
                    n5036 = local write "Hexapod COMM"(w3749) -> ()
                    n5037 = Set Menu Item Info(6:w3749, 7:"com_Secondaire Actif" ("menu tag"), 8:w3716, 11:w3717) -> (0:w3713:errorcluster, 3:w3714:refnum<k9>)  [unwired: 3 in]
                    n5038 = Set Menu Item Info(7:"main_Tables de guidage" ("menu tag"), 8:w3713, 9:w3751, 11:w3714) -> (0:w3722:errorcluster, 3:w3725:refnum<k9>)  [unwired: 3 in]
                    n5039 = Set Menu Item Info(7:"main_Secondaire Actif" ("menu tag"), 8:w3722, 9:w3749, 11:w3725) -> (0:w3718:errorcluster, 3:w3724:refnum<k9>)  [unwired: 3 in]
                    n5040 = Set Menu Item Info(7:"main_Caméra de référence" ("menu tag"), 8:w3718, 9:w3750, 11:w3724) -> (0:w3719:errorcluster, 3:w3720:refnum<k9>)  [unwired: 3 in]
                    n5041 = Set Menu Item Info(7:"main_Télescope" ("menu tag"), 8:w3719, 9:w3748, 11:w3720) -> (0:w3721:errorcluster, 3:w3723:refnum<k9>)  [unwired: 3 in]
                    n5042 = Set Menu Item Info(6:w3752, 7:"main_Roue à filtres" ("menu tag"), 8:w3721, 11:w3723) -> ()  [unwired: 3 in, 2 out]
                  }
                }
              }
              frame #2 {
                n5043 = Tick Count (ms)() -> (millisecond timer value=w3757:u32)
                n5044 = Subtract(x=w3757, y=w3756) -> (x-y=→"CommCheck":u32)
              }
              frame #3 {
                # "Update les registres d'état"
                n5045 = local read "TCS VRN"() -> (w3761:refnum<visa-resource-name>)
                n5046 = control-ref of="TCS actif"() -> (w3759:refnum<vi>)
                n5047 = local read "TCSMute"() -> (w3758:bool)
                n5048 = Tick Count (ms)() -> (millisecond timer value=w3774:u32)
                n5049 = case shown="Faux" w3758 {
                  tunnel: [w3790 w3792] -> w3781
                  tunnel: [w3789 w3792] -> w3780
                  tunnel: [w3788 w3792] -> w3779
                  tunnel: [w3787 w3792] -> w3778
                  tunnel: w3761 -> [w3785 w3791]
                  tunnel: [w3783 w3791] -> w3760
                  tunnel: w3759 -> [w3782 _]
                  frame False {
                    n5050 = call "EXCOM-26.vi"("VRN IN"=w3785, "Bool Refnum"=w3782) -> ("STATL"=w3790:bool[], "STATH"=w3789:bool[], "VRN OUT"=w3784:refnum<visa-resource-name>, "STATEX"=w3787:bool[], "STATLH"=w3788:bool[], "Error OUT"=w3786:errorcluster)  [unwired: 7 in, 1 out]
                    n5051 = call-poly "PolyCommError.vi"("VISA IN"=w3784, "error IN"=w3786) -> ("VISA OUT"=w3783:refnum<visa-resource-name>)  [unwired: 11 in, 2 out]
                  }
                  frame True {
                    w3792 = bool[] [] ("STATL")
                  }
                }
                n5052 = Subtract(x=w3774, y=w3773) -> (x-y=→"Wait4Flag":u32)
                n5053 = local write "Indicateur d'état"("Lecture du statut de TCS" ("Indicateur d'état")) -> ()
                n5054 = local read "Slewing"() -> (w3777:bool)
                n5055 = local read "Focus slew"() -> (w3776:bool)
                n5056 = local write "TCS VRN"(w3760) -> ()
                n5057 = flat-sequence {
                  tunnel: "Setting" -> [w3794]
                  tunnel: w3776 -> [w3795]
                  tunnel: w3777 -> [w3796]
                  tunnel: w3778 -> [w3797]
                  tunnel: w3779 -> [w3798]
                  tunnel: w3780 -> [w3799]
                  tunnel: w3781 -> [w3800]
                  tunnel: [w3800] -> w3770
                  tunnel: [w3799] -> w3769
                  tunnel: [w3798] -> w3768
                  tunnel: [w3797] -> w3767
                  tunnel: [w3796] -> w3766
                  tunnel: [w3795] -> w3765
                  tunnel: [w3794] -> w3764
                  tunnel: [w3793] -> w3763
                  tunnel: w3770 -> [w3834]
                  tunnel: w3769 -> [w3833]
                  tunnel: w3768 -> [w3832]
                  tunnel: w3767 -> [w3831]
                  tunnel: w3766 -> [w3830]
                  tunnel: w3765 -> [w3829]
                  tunnel: w3764 -> [w3828]
